vi "LVClasse_Phase Write Intensity.vi"(8 "error in (no error)":errorcluster, 10 "Intensity":i32, 11 "Intensity in":refnum<class "Intensity.lvclass">) -> (0 "error out":errorcluster, 3 "Intensity out":refnum<class "Intensity.lvclass">)   [LabVIEW 2020, in "Intensity.lvclass"]
uses:
  Intensity.lvclass
  Intensity.lvclass/Intensity.ctl
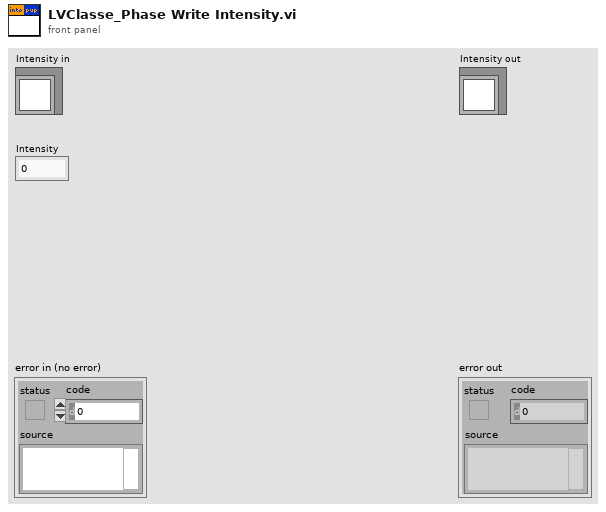
[diagram p1: front panel]
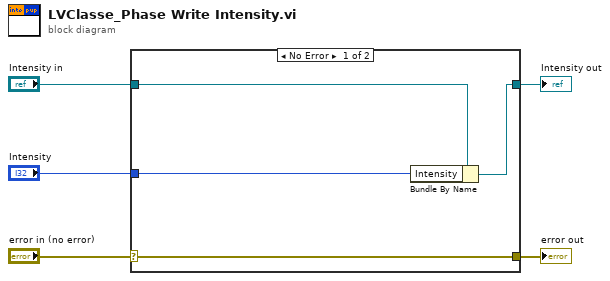
[diagram p0: block diagram]
diagram:
  n1 = case shown="No Error" "error in (no error)" {
    selector: "error in (no error)" -> [w9 w10]
    tunnel: [w9 w10] -> w4
    tunnel: [w7 w11] -> w2
    tunnel: "Intensity in" -> [w8 w11]
    tunnel: "Intensity" -> [w6 _]
    frame No Error {
      n2 = Bundle By Name(cluster=w8, "Intensity"=w6) -> (w7:refnum<class "Intensity.lvclass">)
    }
    frame Error {
    }
  }
  "error out" <- w4
  "Intensity out" <- w2
